vi "add_boolean_control.vi"(8 "error in (no error)":errorcluster, 9 "Single Control Spec":T1, 10 "BD Position":cluster{"Left":i32, "Top":i32}, 11 "VI Ref In":refnum<vi>) -> (0 "error out":errorcluster, 2 "Control Ref Out":refnum<vi>, 3 "VI Ref Out":refnum<vi>)   [LabVIEW 2018]
uses:
  TypeDefinitions/single_control_spec.ctl
  TypeDefinitions/control_data_type.ctl
  TypeDefinitions/control_class.ctl
  TypeDefinitions/ring_string_and_value.ctl
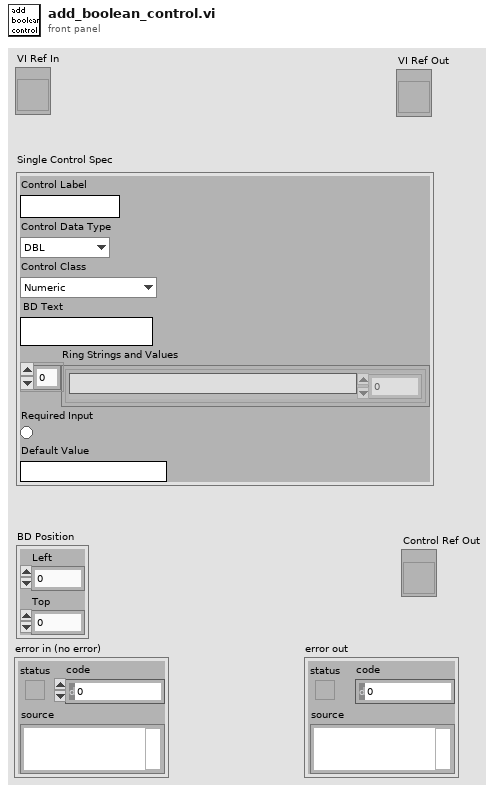
[diagram p1: front panel]
types:
  T1 = typedef "single_control_spec.ctl" = cluster{"Control Label":string, "Control Data Type":T2, "Control Class":T3, "BD Text":string, "Ring Strings and Values":T4[], "Required Input":bool, "Default Value":string}
  T2 = typedef "control_data_type.ctl" = enum16{"DBL", "I32", "Boolean", "String", "U16", "U32", "EXT", "SGL", "I16", "U8", "I8", "I64", "U64", "Waveform", "Reference", "Variant", "Cluster"}
  T3 = typedef "control_class.ctl" = enum16{"Numeric", "Vertical Slide Switch", "Text Ring", "String", "Array", "VISAName", "WaveformGraph", "Cluster"}
  T4 = typedef "ring_string_and_value.ctl" = cluster{"String":string, "Value":dbl}
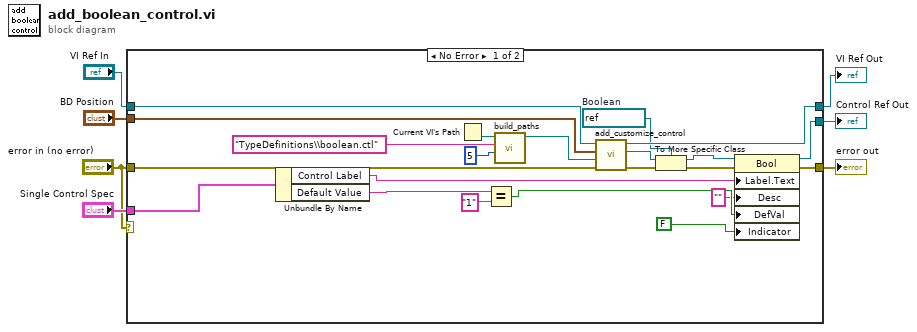
[diagram p0: block diagram]
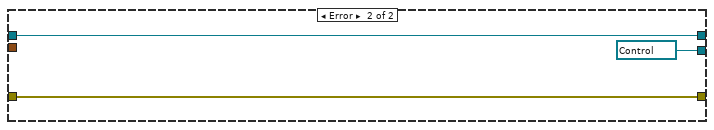
[diagram p2: hidden frame]
diagram:
  n1 = case shown="No Error" "error in (no error)" {
    tunnel: "VI Ref In" -> [w24 w30]
    tunnel: "error in (no error)" -> [w23 w32]
    tunnel: "Single Control Spec" -> [w28 _]
    tunnel: [w27 refnum<vi> refnum ("Ctl Refnum")] -> w5
    tunnel: [w26 w32] -> w4
    tunnel: [w25 w30] -> w2
    tunnel: "BD Position" -> [w22 _]
    frame No Error {
      w10 = refnum<vi> refnum  # Boolean
      n2 = Unbundle By Name(w28) -> ("Control Label"=w8:string, "Default Value"=w21:string)
      n3 = Current VI's Path() -> (path=w16:path)
      n4 = Equal?(x=w21, y="1") -> (x = y?=w18:bool)
      n5 = call "build_paths.vi"("Numeric"=5, "name or relative path"="TypeDefinitions\\boolean.ctl", "path"=w16) -> ("appended path"=w14:path)  [unwired: 6 out]
      n6 = call "add_customize_control.vi"("error in"=w23, "Control Path"=w14, "Control Position on BD"=w22, "VI Ref In"=w24) -> ("error out"=w11:errorcluster, "Ctl Refnum"=w12:refnum<vi>, "VI Ref Out"=w25:refnum<vi>)  [unwired: 5 out]
      n7 = To More Specific Class(target class=w10, reference=w12, error in=w11) -> (specific class reference=w20:refnum<vi>, error out=w19:errorcluster)
      n8 = property class="Bool"(reference=w20, error in=w19, "Label.Text"=w8, "Desc"="" ("Description"), "DefVal"=w18, "Indicator"=FALSE) -> (reference out=w27:refnum<vi>, error out=w26:errorcluster)
    }
    frame Error {
    }
  }
  "VI Ref Out" <- w2
  "Control Ref Out" <- w5
  "error out" <- w4
